vi "SendBinary.vi"(4 "mask":u32=513 format="%.0x", 5 "payload":string, 6 "error in":errorcluster, 9 "connection ID":refnum<k5>) -> (0 "error out":errorcluster, 3 "connection ID out":refnum<k5>)   [LabVIEW 2014, in "Websocket.lvlib"]
uses:
  Websocket.lvlib
  WebsocketFrameTypes_TD.ctl
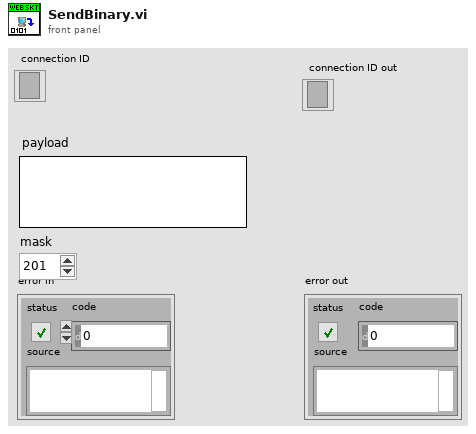
[diagram p1: front panel]
types:
  T1 = typedef "Websocket.lvlib/WebsocketFrameTypes_TD.ctl" = enum8{"Continuation", "Text", "Binary", "Reserved 1", "Reserved 2", "Reserved 3", "Reserved 4", "Reserved 5", "Close", "Ping", "Pong", "Reserved 6", "Reserved 7", "Reserved 8", "Reserved 9", "Reserved 10"}
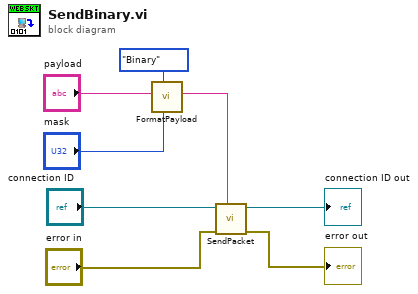
[diagram p0: block diagram]
diagram:
  n1 = call "FormatPayload.vi"("mask value"="mask", "opcode"=WebsocketFrameTypes_TD."Binary", "payload"="payload") -> ("packet"=w1:string)  [unwired: 8 in]
  n2 = call "SendPacket.vi"("payload"=w1, "error in"="error in", "connection ID"="connection ID") -> ("error out"=→"error out":errorcluster, "connection ID out"=→"connection ID out":refnum<k5>)  [unwired: 5 in]
